vi "Controls_de-activate.vi"(0 "Boolean":bool=TRUE, 1 "Array of references":refnum<vi>[](array[refnum])) -> ()   [LabVIEW 2015]
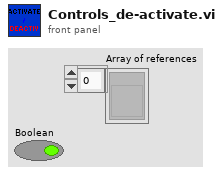
[diagram p1: front panel]
types:
  T1 = enum8{"Enabled", "Disabled", "Disabled and Grayed Out"}
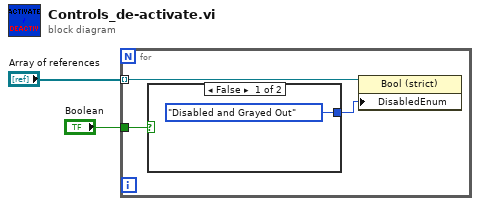
[diagram p0: block diagram]
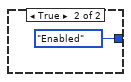
[diagram p2: hidden frame]
diagram:
  n1 = for {
    tunnel: "Array of references" -> [w5] mode=indexing
    tunnel: "Boolean" -> [w3]
    n2 = case shown="False" w3 {
      tunnel: [T1."Disabled and Grayed Out" ("Disabled") T1."Enabled" ("Disabled")] -> w4
      frame False {
      }
      frame True {
      }
    }
    n3 = property class="Bool (strict)"(reference=w5, "DisabledEnum"=w4) -> ()  [unwired: 1 in, 2 out]
  }
